vi "groundwater log header.vi"(5 "Worksheet Names":string[](array[string]), 7 "Groundwater Header":T1, 8 "error in (no error)":errorcluster, 11 "NI_report in":refnum<class "NI_report.lvclass">) -> (0 "error out":errorcluster, 3 "NI_report out":refnum<class "NI_report.lvclass">)   [LabVIEW 2016]
uses:
  <vilib>/Utility/NIReport.llb/NI_report.lvclass
  Groundwater header.ctl
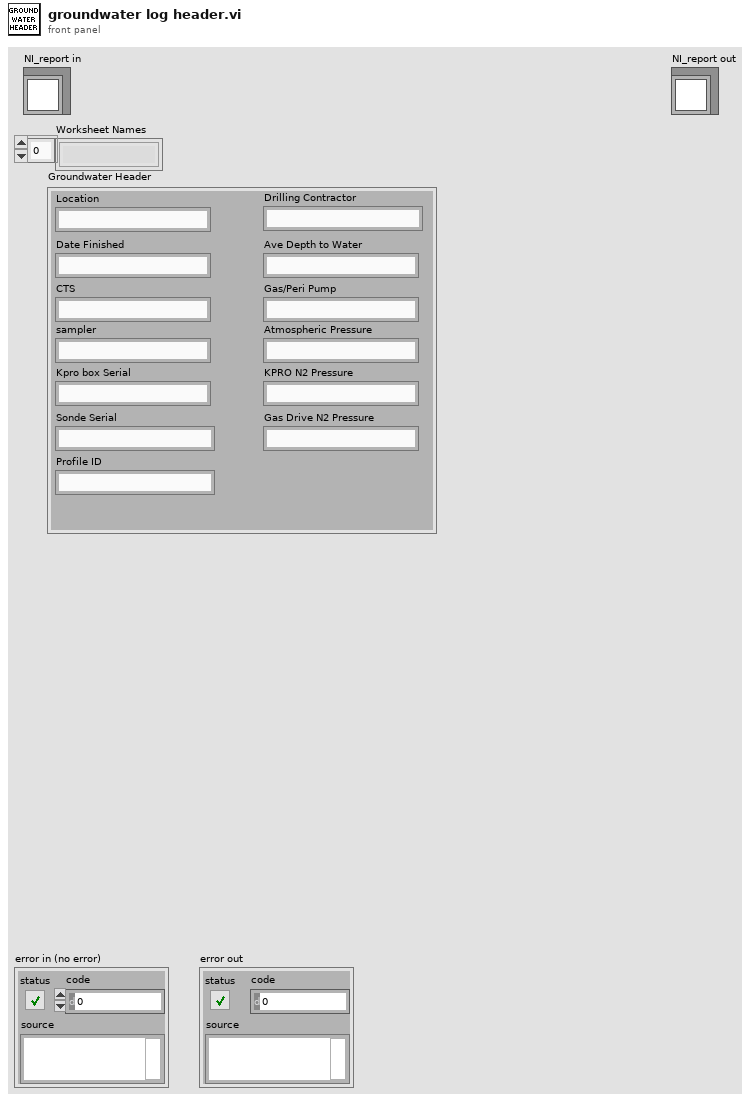
[diagram p1: front panel]
types:
  T1 = typedef "Groundwater header.ctl" = cluster{"Location":string, "Date Finished":string, "CTS":string, "sampler":string, "Kpro box Serial ":string, "Sonde Serial":string, "Drilling Contractor":string, "Ave Depth to Water":string, "Gas/Peri Pump":string, "Atmospheric Pressure":string, "KPRO N2 Pressure":string, "Gas Drive N2 Pressure":string, "Profile ID":string}
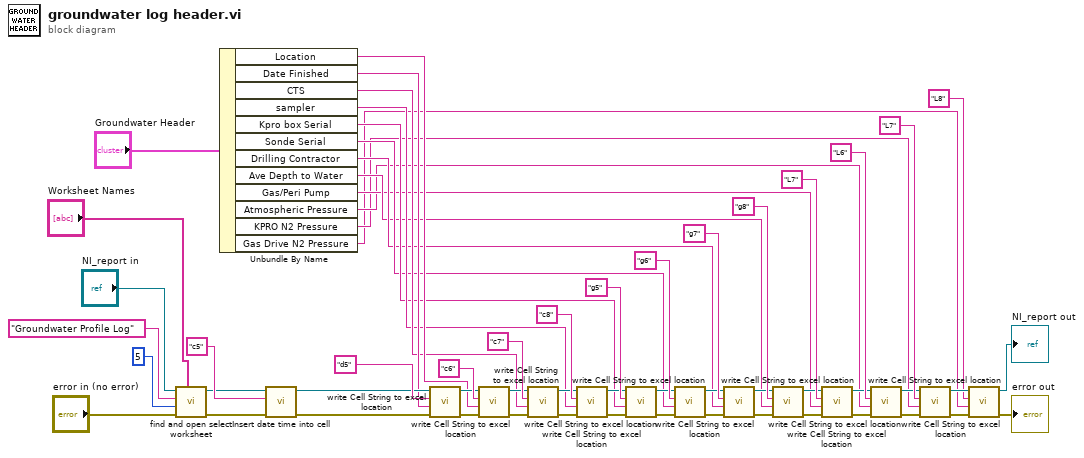
[diagram p0: block diagram]
diagram:
  n1 = call "find and open select worksheet.vi"("Worksheet Names"="Worksheet Names", "error in (no error)"="error in (no error)", "milliseconds to wait"=u32 5, "Worksheet Name in"="Groundwater Profile Log" ("Worksheet Name"), "NI_report in"="NI_report in") -> ("error out"=w19:errorcluster, "NI_report out"=w18:refnum<class "NI_report.lvclass">)  [unwired: 4 in, 1 out]
  n2 = Unbundle By Name("Groundwater Header") -> ("Location"=w11:string, "Date Finished"=w12:string, "CTS"=w10:string, "sampler"=w9:string, "Kpro box Serial"=w8:string, "Sonde Serial"=w7:string, "Drilling Contractor"=w6:string, "Ave Depth to Water"=w5:string, "Gas/Peri Pump"=w4:string, "Atmospheric Pressure"=w3:string, "KPRO N2 Pressure"=w2:string, "Gas Drive N2 Pressure"=w1:string)
  n3 = call "Insert date time into cell.vi"("error in (no error)"=w19, "Date/Time Cell"="c5", "NI_report in"=w18) -> ("error out"=w22:errorcluster, "NI_report out"=w21:refnum<class "NI_report.lvclass">)  [unwired: 7 in]
  n4 = call "write Cell String to excel location.vi"("error in (no error)"=w22, "input string"=w12, "cell's name"="d5", "NI_report in"=w21) -> ("error out"=w23:errorcluster, "NI_report out"=w24:refnum<class "NI_report.lvclass">)  [unwired: 6 in]
  n5 = call "write Cell String to excel location.vi"("error in (no error)"=w23, "input string"=w11, "cell's name"="c6", "NI_report in"=w24) -> ("error out"=w25:errorcluster, "NI_report out"=w26:refnum<class "NI_report.lvclass">)  [unwired: 6 in]
  n6 = call "write Cell String to excel location.vi"("error in (no error)"=w25, "input string"=w10, "cell's name"="c7", "NI_report in"=w26) -> ("error out"=w27:errorcluster, "NI_report out"=w28:refnum<class "NI_report.lvclass">)  [unwired: 6 in]
  n7 = call "write Cell String to excel location.vi"("error in (no error)"=w27, "input string"=w9, "cell's name"="c8", "NI_report in"=w28) -> ("error out"=w29:errorcluster, "NI_report out"=w31:refnum<class "NI_report.lvclass">)  [unwired: 6 in]
  n8 = call "write Cell String to excel location.vi"("error in (no error)"=w29, "input string"=w8, "cell's name"="g5", "NI_report in"=w31) -> ("error out"=w30:errorcluster, "NI_report out"=w32:refnum<class "NI_report.lvclass">)  [unwired: 6 in]
  n9 = call "write Cell String to excel location.vi"("error in (no error)"=w30, "input string"=w7, "cell's name"="g6", "NI_report in"=w32) -> ("error out"=w40:errorcluster, "NI_report out"=w41:refnum<class "NI_report.lvclass">)  [unwired: 6 in]
  n10 = call "write Cell String to excel location.vi"("error in (no error)"=w40, "input string"=w6, "cell's name"="g7", "NI_report in"=w41) -> ("error out"=w42:errorcluster, "NI_report out"=w43:refnum<class "NI_report.lvclass">)  [unwired: 6 in]
  n11 = call "write Cell String to excel location.vi"("error in (no error)"=w42, "input string"=w5, "cell's name"="g8", "NI_report in"=w43) -> ("error out"=w44:errorcluster, "NI_report out"=w45:refnum<class "NI_report.lvclass">)  [unwired: 6 in]
  n12 = call "write Cell String to excel location.vi"("error in (no error)"=w44, "input string"=w4, "cell's name"="L7", "NI_report in"=w45) -> ("error out"=w48:errorcluster, "NI_report out"=w49:refnum<class "NI_report.lvclass">)  [unwired: 6 in]
  n13 = call "write Cell String to excel location.vi"("error in (no error)"=w48, "input string"=w3, "cell's name"="L6", "NI_report in"=w49) -> ("error out"=w52:errorcluster, "NI_report out"=w53:refnum<class "NI_report.lvclass">)  [unwired: 6 in]
  n14 = call "write Cell String to excel location.vi"("error in (no error)"=w52, "input string"=w2, "cell's name"="L7", "NI_report in"=w53) -> ("error out"=w56:errorcluster, "NI_report out"=w57:refnum<class "NI_report.lvclass">)  [unwired: 6 in]
  n15 = call "write Cell String to excel location.vi"("error in (no error)"=w56, "input string"=w1, "cell's name"="L8", "NI_report in"=w57) -> ("error out"=→"error out":errorcluster, "NI_report out"=→"NI_report out":refnum<class "NI_report.lvclass">)  [unwired: 6 in]
